vi "Get Active.vi"(8 "error in (no error)":errorcluster, 11 "Interaction Splitter in":refnum<class "Interaction Splitter.lvclass">) -> (0 "error out":errorcluster, 2 "Active?":bool, 3 "Interaction Splitter out":refnum<class "Interaction Splitter.lvclass">)   [LabVIEW 2021, in "Interaction Splitter.lvclass"]
doc: "Copyright 2018, Wiebe Walstra, wiebe@carya.nl."
uses:
  Interaction Splitter.lvclass
  Interaction Splitter.lvclass/Interaction Splitter.ctl
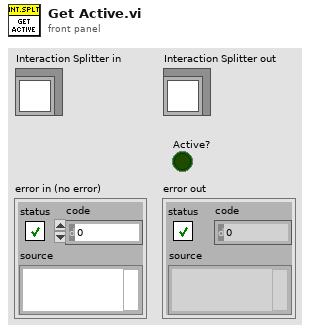
[diagram p1: front panel]
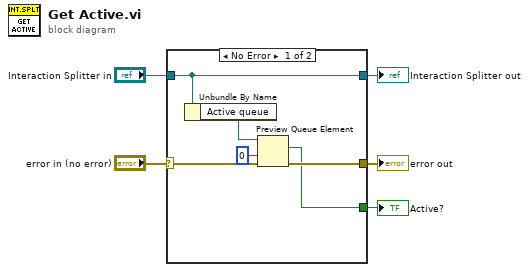
[diagram p0: block diagram]
diagram:
  n1 = case shown="No Error" "error in (no error)" {
    selector: "error in (no error)" -> [w10 w13]
    tunnel: [w9 w13] -> w4
    tunnel: [w11 w12] -> w2
    tunnel: "Interaction Splitter in" -> [w11 w12]
    tunnel: [w6 _] -> w1
    frame No Error {
      n2 = Unbundle By Name(w11) -> ("Active queue"=w8:refnum<queue>)
      n3 = Preview Queue Element(queue=w8, timeout in ms (-1)=0, error in (no error)=w10) -> (element=w6:bool, error out=w9:errorcluster)  [unwired: 2 out]
    }
    frame Error {
    }
  }
  "error out" <- w4
  "Interaction Splitter out" <- w2
  "Active?" <- w1
